vi "Send Done.vi"(5 "Username":string, 6 "Password":string, 7 "Address":string, 8 "Error In":errorcluster) -> (0 "Error Out":errorcluster)   [LabVIEW 2018, in "Tests.lvlib" / "Channel.lvlib"]
uses:
  Channel.lvlib
  <vilib>/addons/_JKI Toolkits/Caraya/classes/Test/Test.lvclass
  <vilib>/addons/_JKI Toolkits/Caraya/classes/Assert/Assert.lvclass
  src/Toolkit/Channel/Channel.lvclass
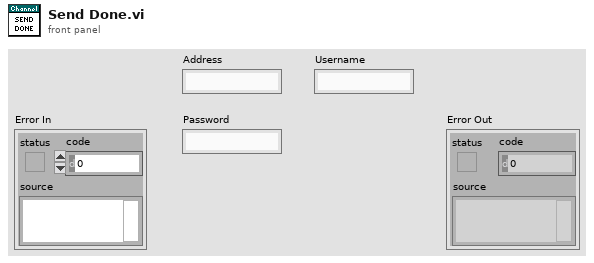
[diagram p1: front panel]
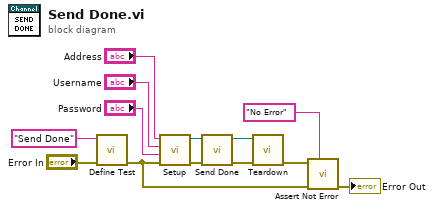
[diagram p0: block diagram]
diagram:
  n1 = call <vilib>:"Define Test.vi"("error in (no error)"="Error In", "Label (VI Title)"="Send Done") -> ("error out"=w10:errorcluster)  [unwired: 9 in]
  n2 = call "Setup.vi"("Error In"=w10, "Password"="Password", "Username"="Username", "Address"="Address") -> ("Error Out"=w2:errorcluster, "Channel"=w5:refnum<class "Channel.lvclass">)  [unwired: 6 in]
  n3 = call "Send Done.vi"("Error In"=w2, "Channel In"=w5) -> ("Error Out"=w3:errorcluster, "Channel Out"=w4:refnum<class "Channel.lvclass">)  [unwired: 8 in]
  n4 = call "Teardown.vi"("Error In"=w3, "Channel"=w4) -> ("Error Out"=w6:errorcluster)  [unwired: 9 in]
  n5 = call <vilib>:"Assert Not Error.vi"("Label"="No Error", "error in (no error)"=w10, "Not Error?"=w6) -> ("error out"=→"Error Out":errorcluster)  [unwired: 8 in]
